vi "SortBundleArray.vi"(1 "Array":T1(array[cluster]) {"End" format="%<%.3X>T"; "Start" format="%<%.3X>T"}) -> (0 "Array 2":T1(array[cluster]) {"End" format="%<%.3X>T"; "Start" format="%<%.3X>T"})   [LabVIEW 2017]
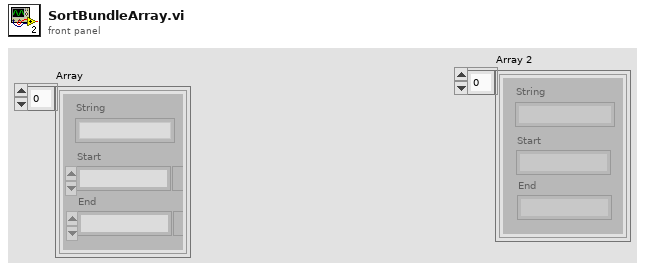
[diagram p1: front panel]
types:
  T1 = cluster{"String":string, "Start":timestamp, "End":timestamp}[]
  T2 = cluster{"String":string, "Start":timestamp, "End":timestamp}
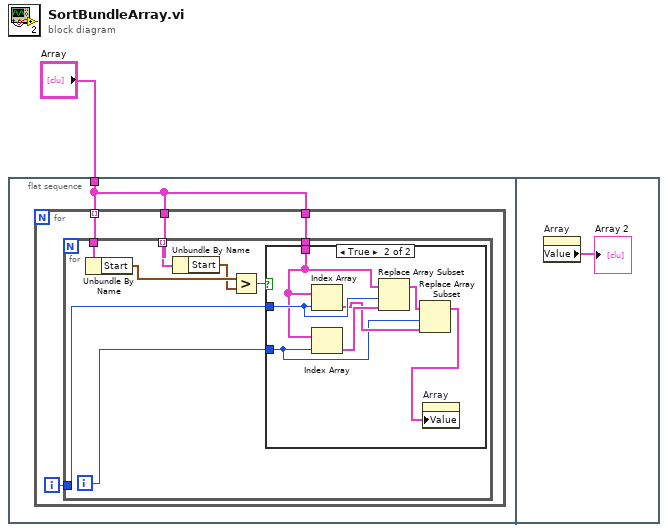
[diagram p0: block diagram]
diagram:
  n1 = flat-sequence {
    tunnel: "Array" -> [w2]
    frame #0 {
      n2 = for {
        tunnel: w2 -> [w5] mode=indexing
        tunnel: w2 -> [w6]
        tunnel: w2 -> [w3]
        i -> [w4]
        n3 = for {
          tunnel: w6 -> [w13] mode=indexing
          tunnel: w5 -> [w14]
          tunnel: w4 -> [w9]
          tunnel: w3 -> [w8]
          i -> [w7]
          n4 = Unbundle By Name(w14) -> ("Start"=w12:timestamp)
          n5 = Unbundle By Name(w13) -> ("Start"=w11:timestamp)
          n6 = Greater?(x=w12, y=w11) -> (0:w10:bool)
          n7 = case shown="True" w10 {
            tunnel: w9 -> [_ w21]
            tunnel: w8 -> [_ w18]
            tunnel: w7 -> [_ w17]
            frame False {
            }
            frame True {
              n8 = Index Array(array=w18, index=w21) -> (element=w19:T2)
              n9 = Index Array(array=w18, index=w17) -> (element=w20:T2)
              n10 = Replace Array Subset(array=w18, new element=w20, index=w21) -> (w16:T1)
              n11 = Replace Array Subset(array=w16, new element=w19, index=w17) -> (w15:T1)
              n12 = property on="Array" class="Arr (strict)"("Value"=w15) -> ()  [unwired: 2 in, 2 out]
            }
          }
        }
      }
    }
    frame #1 {
      n13 = property on="Array" class="Arr (strict)"() -> ("Value"=→"Array 2":T1)  [unwired: 2 in, 2 out]
    }
  }
